vi "GetConfig.vi"(8 "error in (no error)":errorcluster, 11 "reference in":refnum<class "sim_MmW.lvclass">) -> (0 "error out":errorcluster, 2 "String":string, 3 "reference out":refnum<class "sim_MmW.lvclass">)   [LabVIEW 2019, in "sim_MmW.lvclass"]
doc: "Returns actual system configuration as JSON string"
uses:
  sim_MmW.lvclass
  C:/Barkhausen mmWave radar/Development/modules/mmw_instrument/src_LabVIEW/Host/SubVIs/mmWave instrument_class/mmWave instrument.lvclass
  Shared/Config state.ctl
  mmWave instrument_class/System info.ctl
  mmWave instrument_class/System state.ctl
  mmWave instrument_class/Instrument state.ctl
  mmWave instrument_class/Instrument mode.ctl
  mmWave instrument_class/Sync mode.ctl
  mmWave instrument_class/RF port info.ctl
  mmWave instrument_class/mmWave instrument.lvclass
  <vilib>/addons/_JKI.lib/Serialization/JSON/JKI JSON Serialization.lvlib
  Shared/Shared.lvlib
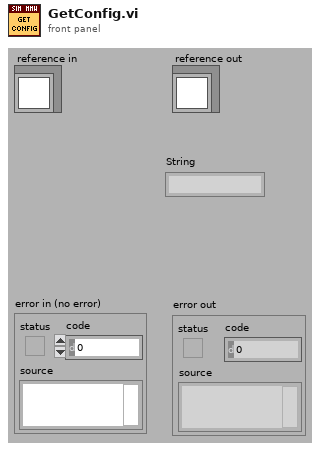
[diagram p1: front panel]
types:
  T1 = typedef "Shared.lvlib/Config state.ctl" = cluster{"system info":T2, "state":T3, "tx":T7, "rx":T7, "versions":cluster{"app":string, "tx fpga":string, "rx fpga":string}}
  T2 = typedef "mmWave instrument.lvclass/System info.ctl" = cluster{"mmw instr":string, "max fs":dbl, "RX/LO1 src":string, "TX/LO1 src":string, "LO2 src":string, "RX LO1 export":bool, "TX LO1 export":bool, "LO2 export":bool, "TX LO1 export level":dbl, "RX LO1 export level":dbl, "LO2 export level":dbl}
  T3 = typedef "mmWave instrument.lvclass/System state.ctl" = cluster{"hw state":T4, "lo sync en":bool, "trig sync en":bool, "mode":T5, "sync":T6, "equalization en":bool}
  T4 = typedef "mmWave instrument.lvclass/Instrument state.ctl" = enum16{"Off", "Initialization", "Configuration", "Running", "Calibration"}
  T5 = typedef "mmWave instrument.lvclass/Instrument mode.ctl" = enum16{"RF", "IF", "BB"}
  T6 = typedef "mmWave instrument.lvclass/Sync mode.ctl" = enum16{"Slave", "Master"}
  T7 = typedef "mmWave instrument.lvclass/RF port info.ctl" = cluster{"fc":dbl, "gain":dbl, "fs":dbl, "trigger delay":dbl}
  T8 = typedef "sim_MmW.lvclass/ObjectAttributes.ctl" = cluster{"RF config":T9, "RX samples":i32, "Downloaded Bursts":map{string, refnum<class "mmWave data.lvclass">}, "TX Fs":dbl, "RX Fs":dbl, "burst sequence":string[], "Burst mode":T10}
  T9 = typedef "mmWave HW Control.lvlib/HW TXRX RF config cluster.ctl" = cluster{"TX.Frequency":dbl, "TX.Gain":dbl, "TX.mmWave adapter":string, "RX.Frequency":dbl, "RX.Gain":dbl, "RX.mmWave adapter":string}
  T10 = typedef "mmWave instrument.lvclass/BurstMode.ctl" = enum16{"burst", "continuous"}
  T11 = typedef "mmWave instrument.lvclass/ObjectAttributes.ctl" = cluster{"mode":T5, "instr state":T4, "Max Fs":dbl, "Equalization coeff":cdb[], "LO sync en":bool, "Trig sync en":bool, "LO sources":T12, "LO Export":T13, "Fc.range":cluster{"min":dbl, "max":dbl}, "Sync mode":T6, "equalization en":bool, "sequence":string[]}
  T12 = typedef "mmWave HW Control.lvlib/LO sources.ctl" = cluster{"RX/LO1 src":string, "TX/LO1 src":string, "LO2 src":string}
  T13 = typedef "mmWave HW Control.lvlib/LO export.ctl" = cluster{"TX LO1 export":bool, "TX LO1 export level":dbl, "RX LO1 export":bool, "RX LO1 export level":dbl, "LO2 export":bool, "LO2 export level":dbl}
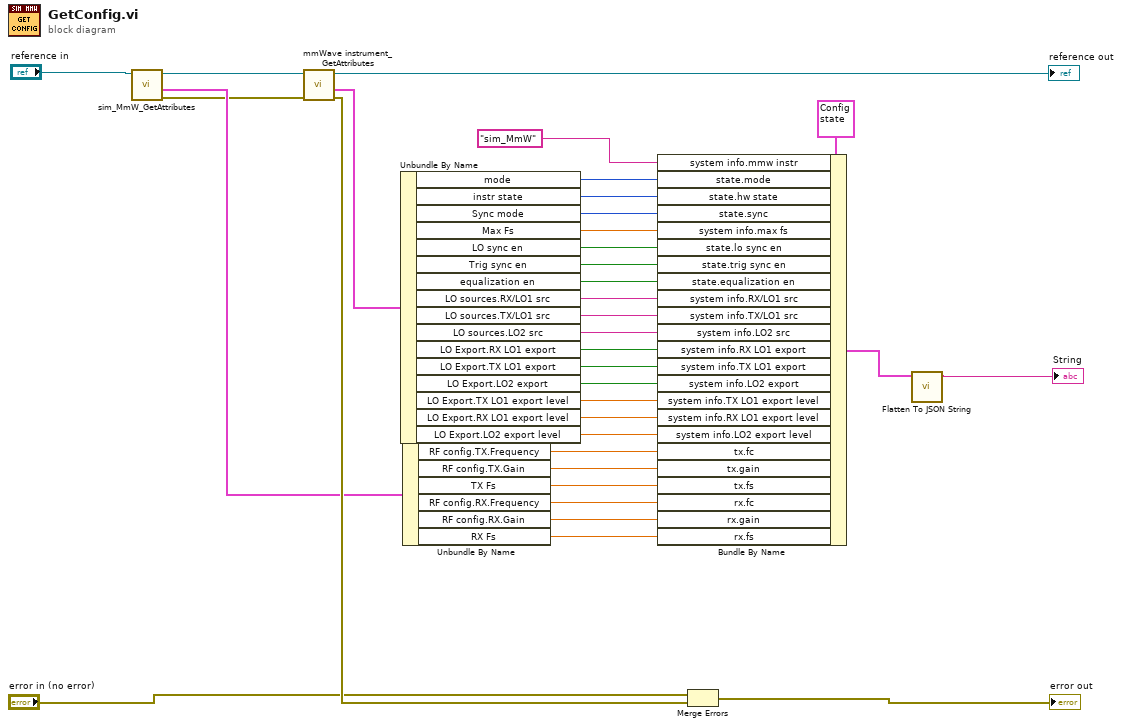
[diagram p0: block diagram]
diagram:
  n1 = call "sim_MmW_GetAttributes.vi"("reference in"="reference in") -> ("error out"=w6:errorcluster, "attributes"=w31:T8, "reference out"=w30:refnum<class "sim_MmW.lvclass">)  [unwired: 7 in, 1 out]
  n2 = call "mmWave instrument_GetAttributes.vi"("error in (no error)"=w6, "reference in"=w30) -> ("error out"=w35:errorcluster, "attributes"=w29:T11, "reference out"=→"reference out":refnum<class "sim_MmW.lvclass">)  [unwired: 6 in, 1 out]
  n3 = Unbundle By Name(w29) -> ("mode"=w27:T5, "instr state"=w26:T4, "Sync mode"=w2:T6, "Max Fs"=w25:dbl, "LO sync en"=w24:bool, "Trig sync en"=w23:bool, "equalization en"=w1:bool, "LO sources.RX/LO1 src"=w22:string, "LO sources.TX/LO1 src"=w21:string, "LO sources.LO2 src"=w20:string, "LO Export.RX LO1 export"=w19:bool, "LO Export.TX LO1 export"=w18:bool, "LO Export.LO2 export"=w17:bool, "LO Export.TX LO1 export level"=w16:dbl, "LO Export.RX LO1 export level"=w15:dbl, "LO Export.LO2 export level"=w14:dbl)
  n4 = Unbundle By Name(w31) -> ("RF config.TX.Frequency"=w13:dbl, "RF config.TX.Gain"=w12:dbl, "TX Fs"=w11:dbl, "RF config.RX.Frequency"=w10:dbl, "RF config.RX.Gain"=w9:dbl, "RX Fs"=w8:dbl)
  n5 = Bundle By Name(cluster=T1 {"system info"={"mmw instr"="", "max fs"=0.0, "RX/LO1 src"="", "TX/LO1 src"="", "LO2 src"="", "RX LO1 export"=FALSE, "TX LO1 export"=FALSE, "LO2 export"=FALSE, "TX LO1 export level"=0.0, "RX LO1 export level"=0.0, "LO2 export level"=0.0}, "state"={"hw state"=enum."Off", "lo sync en"=FALSE, "trig sync en"=FALSE, "mode"=enum."RF", "sync"=enum."Slave", "equalization en"=FALSE}, "tx"={"fc"=0.0, "gain"=0.0, "fs"=0.0, "trigger delay"=0.0}, "rx"={"fc"=0.0, "gain"=0.0, "fs"=0.0, "trigger delay"=0.0}, "versions"={"app"="", "tx fpga"="", "rx fpga"=""}} ("Transciever config"), "system info.mmw instr"="sim_MmW" ("sistem info.mmw instr"), "state.mode"=w27, "state.hw state"=w26, "state.sync"=w2, "system info.max fs"=w25, "state.lo sync en"=w24, "state.trig sync en"=w23, "state.equalization en"=w1, "system info.RX/LO1 src"=w22, "system info.TX/LO1 src"=w21, "system info.LO2 src"=w20, "system info.RX LO1 export"=w19, "system info.TX LO1 export"=w18, "system info.LO2 export"=w17, "system info.TX LO1 export level"=w16, "system info.RX LO1 export level"=w15, "system info.LO2 export level"=w14, "tx.fc"=w13, "tx.gain"=w12, "tx.fs"=w11, "rx.fc"=w10, "rx.gain"=w9, "rx.fs"=w8) -> (w7:T1)
  n6 = Merge Errors("error in (no error)", w35) -> (→"error out":errorcluster)
  n7 = call <vilib>:"Flatten To JSON String.vi"("Variant"=w7) -> ("JSON String"=→"String":string)  [unwired: 9 in, 1 out]
